vi "Start Measuring.vi"(8 "error in (no error)":errorcluster, 11 "Coverage Analyzer in":refnum<class "Coverage Analyzer.lvclass">) -> (0 "error out":errorcluster, 3 "Coverage Analyzer out":refnum<class "Coverage Analyzer.lvclass">)   [LabVIEW 2020, in "Coverage Analyzer.lvlib" / "Coverage Analyzer.lvclass"]
uses:
  Coverage Analyzer.lvclass
  Coverage Analyzer.lvclass/Coverage Analyzer.ctl
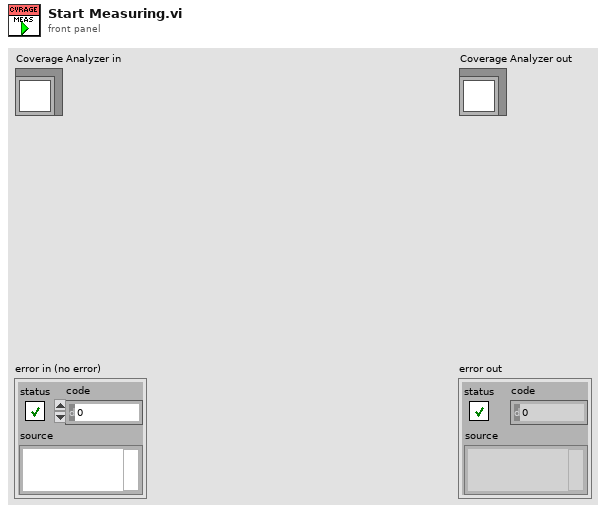
[diagram p1: front panel]
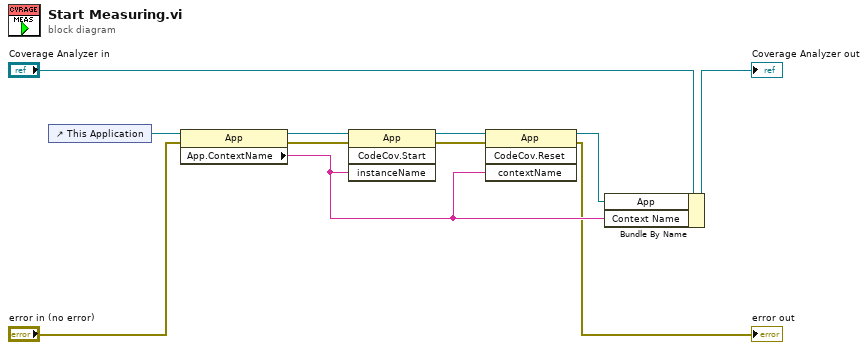
[diagram p0: block diagram]
diagram:
  n1 = control-ref of="This Application"() -> (w10:refnum<vi>)
  n2 = property class="App"(reference=w10, error in="error in (no error)") -> (reference out=w5:refnum<vi>, error out=w9:errorcluster, "App.ContextName"=w6:string)
  n3 = invoke class="App" method="CodeCov.Start"(reference=w5, error in=w9, "instanceName"=w6) -> (reference out=w4:refnum<vi>, error out=w8:errorcluster)  [unwired: 1 in, 2 out]
  n4 = invoke class="App" method="CodeCov.Reset"(reference=w4, error in=w8, "contextName"=w6) -> (reference out=w1:refnum<vi>, error out=→"error out":errorcluster)  [unwired: 1 in, 2 out]
  n5 = Bundle By Name(cluster="Coverage Analyzer in", "App"=w1, "Context Name"=w6) -> (→"Coverage Analyzer out":refnum<class "Coverage Analyzer.lvclass">)
